vi "TDT-Init DAQ (Npts).vi"(0 "AO Fs (Hz)":dbl, 1 "Circuit":string, 2 "AI only":bool, 5 "AI Fs (Hz)":dbl, 7 "Num AO Pts":i32, 9 "Num AO Buffers":i32=2, 11 "error in (no error)":errorcluster, 12 "AO Channels":i32[](array[numeric]), 13 "AI Channels":i32[](array[numeric])=[1, 2]) -> (4 "AO Fs (coerced)":dbl, 6 "AI Fs (coerced)":dbl, 8 "AO npts":i32, 10 "AI npts":i32, 15 "error out":errorcluster)   [LabVIEW 2020]
uses:
  TDT-Signal Bank Action.ctl
  TDT-Globals.vi
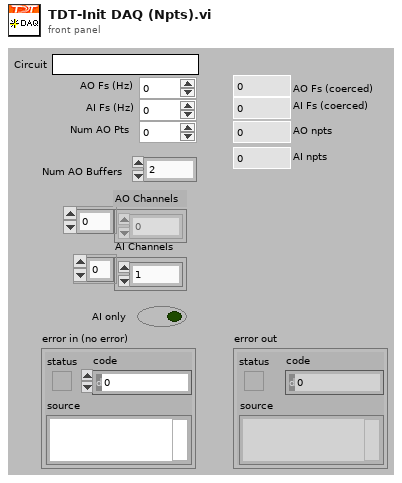
[diagram p1: front panel]
types:
  T1 = typedef "TDT-Signal Bank Action.ctl" = enum16{"Init", "Write", "Read", "Rewrite", "Reset", "Recycle", "Ramp up", "Ramp down", "Zero"}
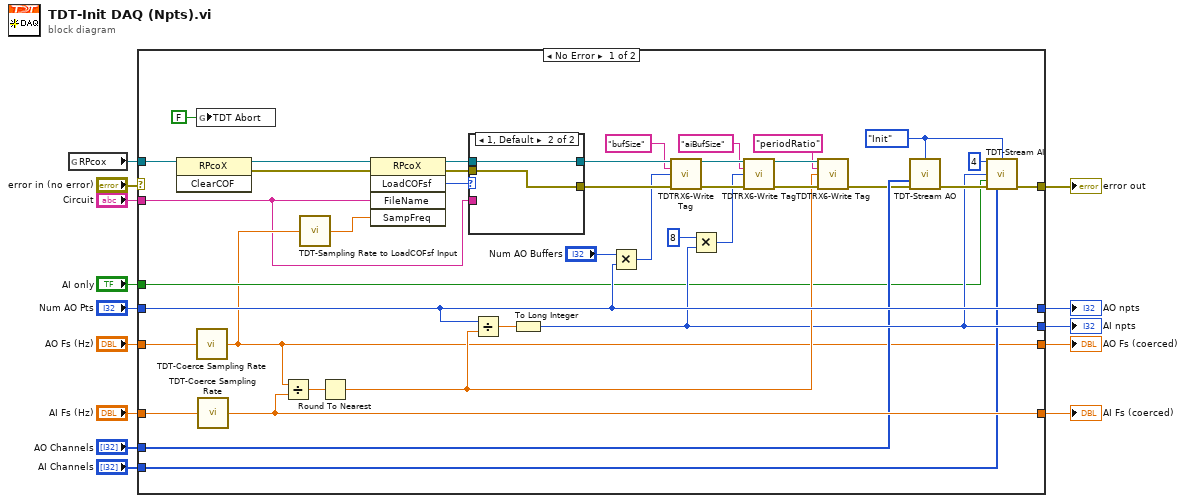
[diagram p0: block diagram]
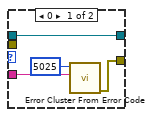
[diagram p2: hidden frame]
diagram:
  n1 = global read "TDT-Globals.vi" "RPcox"() -> (w12:refnum<k7>)
  n2 = case shown="No Error" "error in (no error)" {
    selector: "error in (no error)" -> [_ w60]
    tunnel: [w35 w60] -> w13
    tunnel: w12 -> [w25 _]
    tunnel: "AO Fs (Hz)" -> [w38 _]
    tunnel: "AI Fs (Hz)" -> [w37 _]
    tunnel: "Num AO Pts" -> [w29 _]
    tunnel: [w17 _] -> w8
    tunnel: [w36 _] -> w7
    tunnel: [w29 _] -> w6
    tunnel: [w26 _] -> w5
    tunnel: "AI Channels" -> [w21 _]
    tunnel: "Circuit" -> [w15 _]
    tunnel: "AO Channels" -> [w22 _]
    tunnel: "AI only" -> [w18 _]
    frame No Error {
      w34 = TDT-Signal_Bank_Action."Init" ("Action")
      n3 = invoke class="RPcoX" method="ClearCOF"(reference=w25) -> (reference out=w24:refnum<k7>, error out=w23:errorcluster)  [unwired: 2 in, 1 out]
      n4 = global write "TDT-Globals.vi" "TDT Abort"(FALSE ("TDT Abort")) -> ()
      n5 = call "TDT-Coerce Sampling Rate.vi"("Fs (Hz)"=w38) -> ("Coerced"=w17:dbl)
      n6 = call "TDT-Coerce Sampling Rate.vi"("Fs (Hz)"=w37) -> ("Coerced"=w36:dbl)
      n7 = Divide(x=w17, y=w36) -> (x/y=w39:dbl)
      n8 = call "TDT-Sampling Rate to LoadCOFsf Input.vi"("Sampling rate (Hz)"=w17) -> ("LoadCOFsf Input"=w16:dbl)  [unwired: 14 in]
      n9 = Round To Nearest(number=w39) -> (nearest integer value=w28:dbl)
      n10 = invoke class="RPcoX" method="LoadCOFsf"(reference=w24, error in=w23, "FileName"=w15, "SampFreq"=w16) -> (reference out=w52:refnum<k7>, error out=w51:errorcluster, "LoadCOFsf"=w53:i32)  [unwired: 1 in, 2 out]
      n11 = case shown="1, Default" w53 {
        tunnel: w15 -> [w56 _]
        tunnel: w52 -> [w57 w59]
        tunnel: w51 -> [_ w58]
        tunnel: [w57 w59] -> w50
        tunnel: [w54 w58] -> w49
        frame 0 {
          n12 = call <vilib>:"Error Cluster From Error Code.vi"("error message (\"\")"=w56, "error code (0)"=5025) -> ("error out"=w54:errorcluster)  [unwired: 7 in]
        }
        frame 1, Default {
        }
      }
      n13 = Divide(x=w29, y=w28) -> (x/y=w27:dbl)
      n14 = To Long Integer(number=w27) -> (32bit integer=w26:i32)
      n15 = Multiply(x="Num AO Buffers", y=w29) -> (x*y=w31:i32)
      n16 = call "TDTRX6-Write Tag.vi"("RPcox"=w50, "Name"="bufSize", "Value"=w31, "error in"=w49) -> ("RPcox Out"=w46:refnum<k7>, "error out"=w47:errorcluster)  [unwired: 10 in]
      n17 = Multiply(x=8, y=w26) -> (x*y=w33:i32)
      n18 = call "TDTRX6-Write Tag.vi"("RPcox"=w46, "Name"="aiBufSize", "Value"=w33, "error in"=w47) -> ("RPcox Out"=w43:refnum<k7>, "error out"=w44:errorcluster)  [unwired: 10 in]
      n19 = call "TDTRX6-Write Tag.vi"("RPcox"=w43, "Name"="periodRatio", "Value"=w28, "error in"=w44) -> ("error out"=w19:errorcluster)  [unwired: 10 in, 1 out]
      n20 = call "TDT-Stream AO.vi"("Action"=w34, "Chans"=w22, "error in (no error)"=w19) -> ("error out"=w41:errorcluster)  [unwired: 12 in]
      n21 = call "TDT-Stream AI.vi"("#Inputs"=4, "Action"=w34, "Pts Per Read"=w26, "AI only"=w18, "error in (no error)"=w41, "AI Channels"=w21) -> ("error out"=w35:errorcluster)  [unwired: 8 in, 1 out]
    }
    frame Error {
    }
  }
  "error out" <- w13
  "AO Fs (coerced)" <- w8
  "AI Fs (coerced)" <- w7
  "AO npts" <- w6
  "AI npts" <- w5
